vi "Create Pattern TXT.vi"(8 "error in (no error)":errorcluster, 9 "ChipID":u8, 10 "Frame_Data":T1 {"Data" format="%x"; "Start_Addr" format="%x"}, 11 "BML_Root in":refnum<class "BML_Root.lvclass">) -> (0 "error out":errorcluster, 3 "BML_Root out":refnum<class "BML_Root.lvclass">)   [LabVIEW 2016, in "BML_Root.lvclass"]
uses:
  BML_Root.lvclass
  Config_Read/Frame_Data.ctl
  Config_Read/OperationMode.ctl
  Config_Read/BurstLength.ctl
  Config_Read/RW_Option.ctl
  Config_Read/Config_Read.lvclass
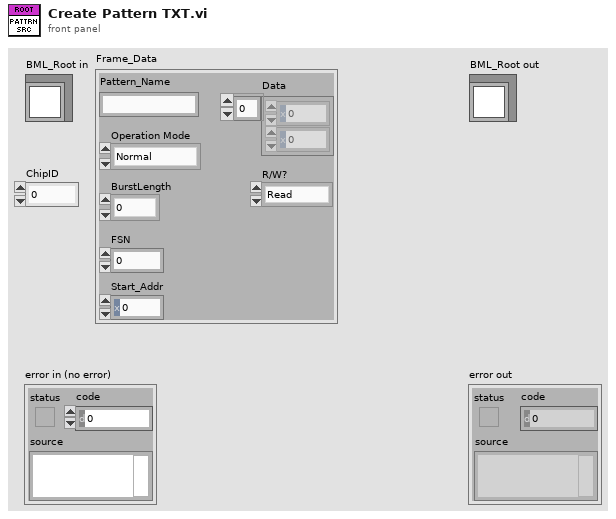
[diagram p1: front panel]
types:
  T1 = typedef "Config_Read.lvclass/Frame_Data.ctl" = cluster{"Pattern_Name":string, "Operation Mode":T2, "BurstLength":T3, "FSN":u8, "Start_Addr":u16, "Data":u8[], "R/W?":T4}
  T2 = typedef "Config_Read.lvclass/OperationMode.ctl" = enum8{"Normal", "ImmeEffect", "InitSlaveID", "LoadData"}
  T3 = typedef "Config_Read.lvclass/BurstLength.ctl" = enum8{"0", "2", "3", "4", "5", "8", "16", "32"}
  T4 = typedef "Config_Read.lvclass/RW_Option.ctl" = enum16{"Read", "Write", "R/W"}
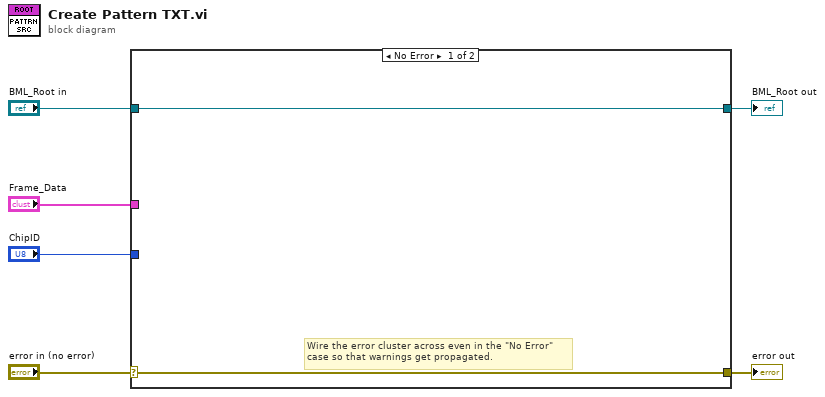
[diagram p0: block diagram]
diagram:
  n1 = case shown="No Error" "error in (no error)" {
    selector: "error in (no error)" -> [w7 w10]
    tunnel: [w7 w10] -> w5
    tunnel: [w8 w9] -> w3
    tunnel: "BML_Root in" -> [w8 w9]
    tunnel: "Frame_Data" -> [_ _]
    tunnel: "ChipID" -> [_ _]
    frame No Error {
      # "Wire the error cluster across even in the \"No Error\"\ncase so that warnings get propagated."
    }
    frame Error {
    }
  }
  "error out" <- w5
  "BML_Root out" <- w3
